vi "usb relay exit.vi"(8 "error in (no error)":errorcluster caption="entrée d'erreur (pas d'erreur)") -> (0 "error out":errorcluster caption="sortie d'erreur", 3 "function return":i32)   [LabVIEW 2020, in "usb_relay_device.lvlib"]
doc: "int EXPORT_API usb_relay_exit(void);"
uses:
  usb_relay_device.lvlib
  usb_relay_device.dll
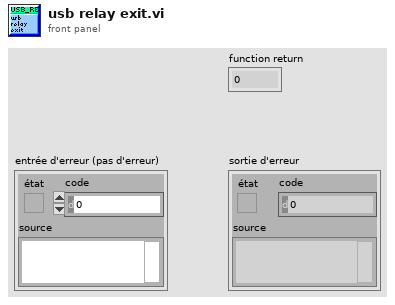
[diagram p1: front panel]
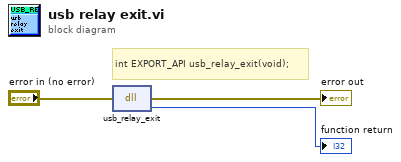
[diagram p0: block diagram]
diagram:
  # "int EXPORT_API usb_relay_exit(void);"
  n1 = dll-call lib="C:/Users/ngarcin/OneDrive - Altyor/Standard TB/Class/Relay_Board/Relay_Board usb_Relay_device/usb_relay_device/usb_relay_device.*" fn="usb_relay_exit"(error in="error in (no error)") -> (error out=→"error out":errorcluster, "type de retour"=→"function return":i32)  [unwired: 2 in, 1 out]
